vi "Method One Numeric Argument.vi"(8 "error in (no error)":errorcluster, 10 "Numeric":dbl, 11 "Test Interface in":refnum<class "Test Interface.lvclass">) -> (0 "error out":errorcluster, 3 "Test Interface out":refnum<class "Test Interface.lvclass">)   [LabVIEW 2020, in "Test Interface.lvclass"]
uses:
  Test Interface.lvclass
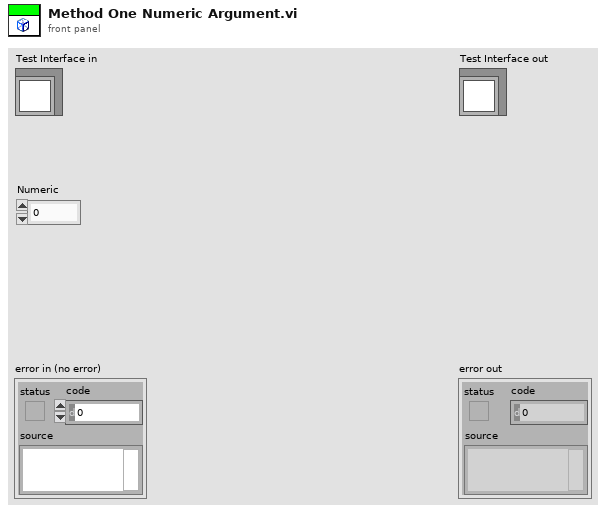
[diagram p1: front panel]
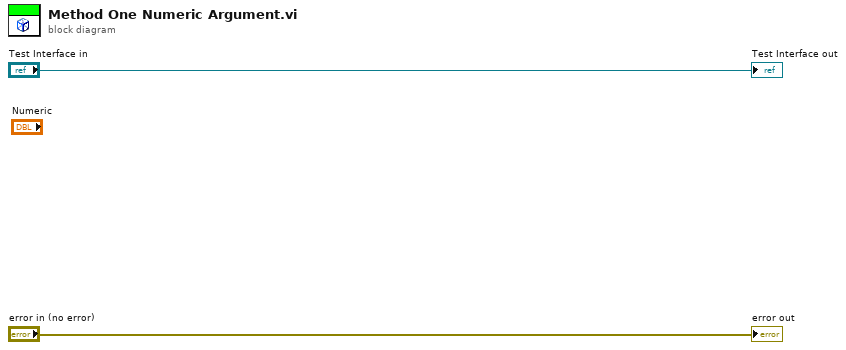
[diagram p0: block diagram]
diagram:
  "error out" <- "error in (no error)"
  "Test Interface out" <- "Test Interface in"
